vi "Update.vi"(10 "Pixel Data in":u32[][](array[numeric]), 11 "Rotating Objects in":refnum<class "Rotating Objects.lvclass">) -> (2 "Pixel Data out":u32[][](array[numeric]), 3 "Rotating Objects out":refnum<class "Rotating Objects.lvclass">)   [LabVIEW 2020, in "Amnesia.lvlib" / "Rotating Objects.lvclass"]
uses:
  Rotating Objects.lvclass
  Scene/Scene.lvclass
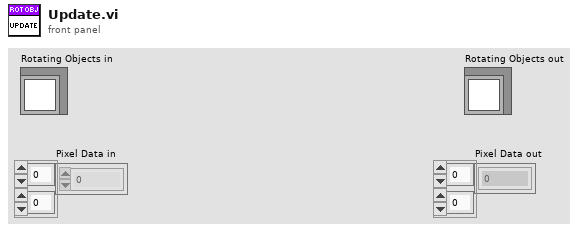
[diagram p1: front panel]
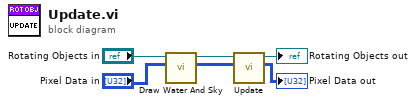
[diagram p0: block diagram]
diagram:
  n1 = call "Draw Water And Sky.vi"("Pixel Data in"="Pixel Data in", "Rotating Objects in"="Rotating Objects in") -> ("Pixel Data out"=w1:u32[][], "Rotating Objects out"=w3:refnum<class "Rotating Objects.lvclass">)  [unwired: 8 in]
  n2 = call-parent "Update.vi"("Pixel Data in"=w1, "Scene in"=w3) -> ("Pixel Data out"=→"Pixel Data out":u32[][], "Scene out"=→"Rotating Objects out":refnum<class "Rotating Objects.lvclass">)  [unwired: 8 in]
